vi "PC_SVG to FDVM with trigger.vi"() -> ()   [LabVIEW 2021]
uses:
  Frequency Domain Measurement/Typedefs/FD Measurements.ctl
  Frequency Domain Measurement/Typedefs/Detected Tones.ctl
  Signal Voltage Generation/Typedefs/Signal Generation Settings.ctl
  Signal Voltage Generation/Typedefs/Generation Types.ctl
  Signal Voltage Generation/Typedefs/Single Tone Settings.ctl
  Signal Voltage Generation/Typedefs/Waveform Type.ctl
  Signal Voltage Generation/Typedefs/Tone Settings.ctl
  Frequency Domain Measurement/Typedefs/Execution Settings.ctl
  Common/Typedefs/Execution Options - Measure.ctl
  Frequency Domain Measurement/Typedefs/Timing & Trigger Settings.ctl
  Frequency Domain Measurement/Typedefs/Timing Settings.ctl
  Signal Voltage Generation/Typedefs/Trigger Settings.ctl
  Frequency Domain Measurement/DAQ_Frequency Domain Measurement.lvlib
  Signal Voltage Generation/DAQ_Signal Voltage Generation.lvlib
panel:
  out "Generated Voltage Waveforms":waveform(dbl)[](graph)=[{"t0"=timestamp(0 s since 1904-01-01), "dt"=1e-05, "Y"=array[10000 elements]}]
  in  "Signal Generation Settings":T1={"Generation Type"=enum."Multi Tone", "Generation Time (s)"=0.1, "Voltage Offset (v)"=0.0, "Single Tone Settings"={"Waveform Type"=enum."Square Wave", "Frequency (Hz)"=100.0, "Amplitude (V)"=1.0, "Duty Cycle (%)"=50.0}, "Multi Tone Settings"=[{"Frequency (Hz)"=100.0, "Amplitude (V)"=1.0}, {"Frequency (Hz)"=200.0, "Amplitude (V)"=0.3}, {"Frequency (Hz)"=300.0, "Amplitude (V)"=0.05}]} {"Voltage Offset (v)" format="%.2p"; "Generation Time (s)" format="%.2p"; "Multi Tone Settings"."Amplitude (V)" format="%#.2p"; "Multi Tone Settings"."Frequency (Hz)" format="%#.2p"; "Single Tone Settings"."Duty Cycle (%)" format="%#.2p"; "Single Tone Settings"."Amplitude (V)" format="%#.2p"; "Single Tone Settings"."Frequency (Hz)" format="%#.2p"}
  out "Frequency Domain Measurements":T6={"Magnitude RMS (dBV)"=[{"f0"=0.0, "df"=10.0, "magnitude"=array[500 elements]}], "Magnitude Peak (dBV)"=[{"f0"=0.0, "df"=10.0, "magnitude"=array[500 elements]}], "Detected Tones"=[{"Frequencies (Hz)"=[99.99975245035697, 199.99921391698715, 299.993454263471], "Amplitudes (V)"=[0.9999999228368428, 0.2999958335995153, 0.049950764634060514]}]} {"Detected Tones"."Amplitudes (V)" format="%.2p"; "Detected Tones"."Frequencies (Hz)" format="%.2p"}
  out "Voltage Waveforms":waveform(dbl)[](graph)=[{"t0"=timestamp(3825153768.619829 s since 1904-01-01), "dt"=9.999999999999999e-05, "Y"=array[1000 elements], "attributes"=variant("NI_ChannelName"=variant(string "Dev1/ai1"), "NI_UnitDescription"=variant(string "Volts"))}]
  out "error out":errorcluster
  # "Frequency (Hz)"
  # "Amplitude (V)"
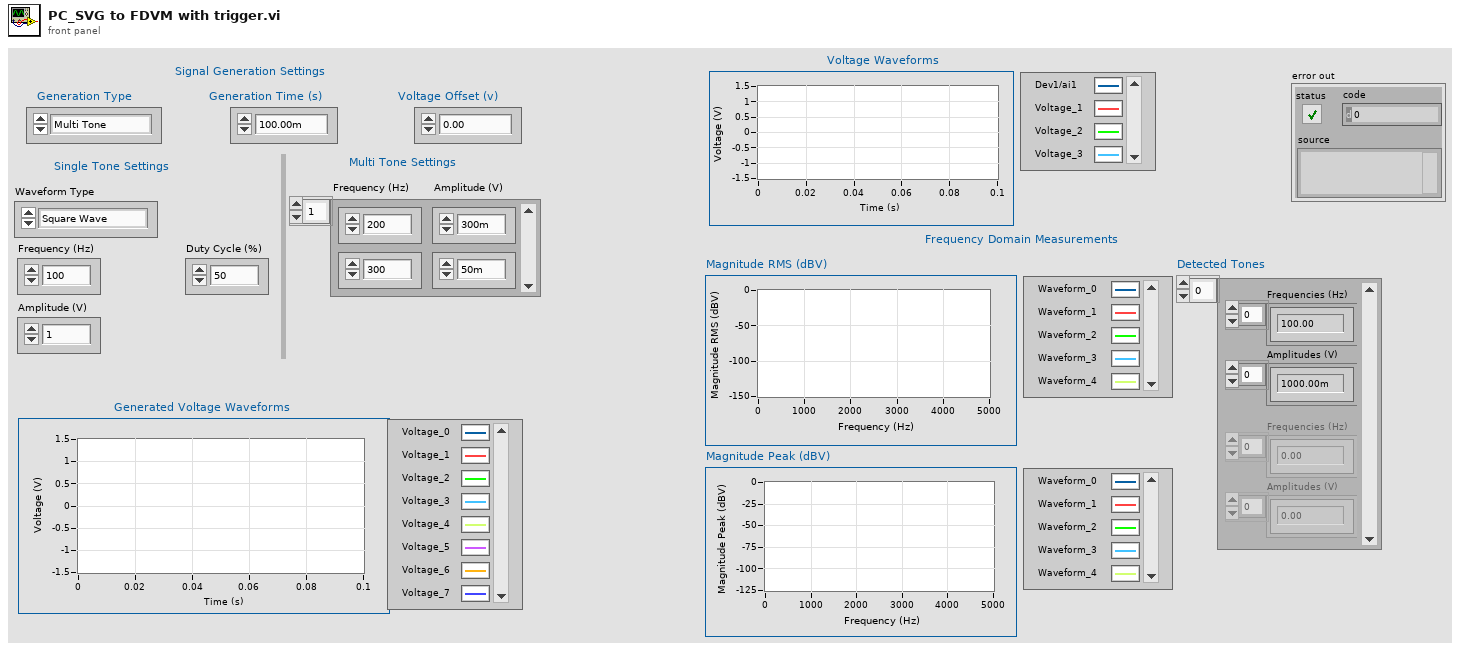
[diagram p1: front panel]
types:
  T1 = typedef "DAQ_Signal Voltage Generation.lvlib/Signal Generation Settings.ctl" = cluster{"Generation Type":T2, "Generation Time (s)":dbl, "Voltage Offset (v)":dbl, "Single Tone Settings":T3, "Multi Tone Settings":T5[]}
  T2 = typedef "DAQ_Signal Voltage Generation.lvlib/Generation Types.ctl" = enum16{"Single Tone", "Multi Tone"}
  T3 = typedef "DAQ_Signal Voltage Generation.lvlib/Single Tone Settings.ctl" = cluster{"Waveform Type":T4, "Frequency (Hz)":dbl, "Amplitude (V)":dbl, "Duty Cycle (%)":dbl}
  T4 = typedef "DAQ_Signal Voltage Generation.lvlib/Waveform Type.ctl" = enum16{"Sine Wave", "Square Wave"}
  T5 = typedef "DAQ_Signal Voltage Generation.lvlib/Tone Settings.ctl" = cluster{"Frequency (Hz)":dbl, "Amplitude (V)":dbl}
  T6 = typedef "DAQ_Frequency Domain Measurement.lvlib/FD Measurements.ctl" = cluster{"Magnitude RMS (dBV)":cluster{"f0":dbl, "df":dbl, "magnitude":dbl[]}[], "Magnitude Peak (dBV)":cluster{"f0":dbl, "df":dbl, "magnitude":dbl[]}[], "Detected Tones":T7[]}
  T7 = typedef "DAQ_Frequency Domain Measurement.lvlib/Detected Tones.ctl" = cluster{"Frequencies (Hz)":dbl[], "Amplitudes (V)":dbl[]}
  T8 = typedef "DAQ_Frequency Domain Measurement.lvlib/Timing & Trigger Settings.ctl" = cluster{"Timing Settings":T9, "Trigger Settings":T10}
  T9 = typedef "DAQ_Frequency Domain Measurement.lvlib/Timing Settings.ctl" = cluster{"Sample Clock Source":tag, "Sample Rate (Hz)":dbl, "Number of Samples":i32, "Sample Timing Engine":enum16{"te0", "te1", "ai", "Auto"}}
  T10 = typedef "DAQ_Signal Voltage Generation.lvlib/Trigger Settings.ctl" = cluster{"Trigger Type":enum16{"No Trigger", "Digital Start"}, "Digital Start Trigger Source":tag, "Digital Start Trigger Edge":i32}
  T11 = typedef "DAQ_Frequency Domain Measurement.lvlib/Execution Settings.ctl" = cluster{"Execution option":T12, "Skip Analysis?":bool}
  T12 = typedef "Execution Options - Measure.ctl" = enum16{"Configure & Measure", "Configure only", "Measure only"}
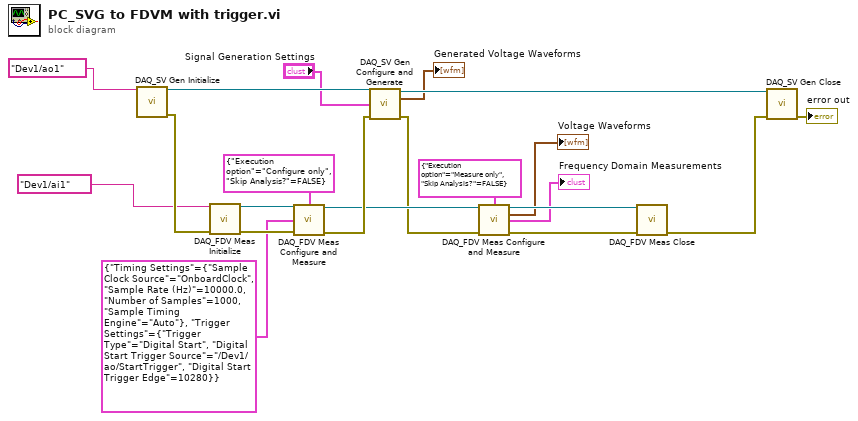
[diagram p0: block diagram]
diagram:
  n1 = call "DAQ_SV Gen Initialize.vi"("Physical Channels"=tag "Dev1/ao1") -> ("DAQmx Task Out"=w21:refnum<k21>, "error out"=w19:errorcluster)  [unwired: 13 in]
  n2 = call "DAQ_FDV Meas Initialize.vi"("Physical Channels"=tag "Dev1/ai1", "error in"=w19) -> ("DAQmx Task Out"=w17:refnum<k21>, "error out"=w18:errorcluster)  [unwired: 12 in]
  n3 = call "DAQ_FDV Meas Configure and Measure.vi"("DAQmx Task In"=w17, "Execution Settings"=T11 {"Execution option"=enum."Configure only", "Skip Analysis?"=FALSE}, "Timing and Trigger Settings"=T8 {"Timing Settings"={"Sample Clock Source"="OnboardClock", "Sample Rate (Hz)"=10000.0, "Number of Samples"=1000, "Sample Timing Engine"=enum."Auto"}, "Trigger Settings"={"Trigger Type"=enum."Digital Start", "Digital Start Trigger Source"="/Dev1/ao/StartTrigger", "Digital Start Trigger Edge"=10280}}, "error in"=w18) -> ("DAQmx Task Out"=w12:refnum<k21>, "error out"=w16:errorcluster)  [unwired: 7 in, 3 out]
  n4 = call "DAQ_SV Gen Configure and Generate.vi"("DAQmx Task In"=w21, "Signal Generation Settings"="Signal Generation Settings", "error in"=w16) -> ("DAQmx Task Out"=w20:refnum<k21>, "Generated Voltage Waveforms"=→"Generated Voltage Waveforms":waveform(dbl)[], "error out"=w10:errorcluster)  [unwired: 10 in]
  n5 = call "DAQ_FDV Meas Configure and Measure.vi"("DAQmx Task In"=w12, "Execution Settings"=T11 {"Execution option"=enum."Measure only", "Skip Analysis?"=FALSE}, "error in"=w10) -> ("DAQmx Task Out"=w11:refnum<k21>, "Voltage Waveforms"=→"Voltage Waveforms":waveform(dbl)[], "Frequency Domain Measurements"=→"Frequency Domain Measurements":T6, "error out"=w9:errorcluster)  [unwired: 8 in, 1 out]
  n6 = call "DAQ_FDV Meas Close.vi"("DAQmx Task In"=w11, "error in"=w9) -> ("error out"=w15:errorcluster)  [unwired: 13 in]
  n7 = call "DAQ_SV Gen Close.vi"("DAQmx Task In"=w20, "error in"=w15) -> ("error out"=→"error out":errorcluster)  [unwired: 13 in]
